vi "Default Instrument Setup.vi"(8 "error in (no error)":errorcluster, 11 "VISA resource name":refnum<visa-resource-name>) -> (0 "error out":errorcluster, 3 "VISA resource name out":refnum<visa-resource-name>)   [LabVIEW 2014, in "GRBLMotionCore.lvlib"]
doc: "This Utility VI sends a default command string to the instrument whenever a new VISA session is opened, or the instrument is reset. Use this VI as a subVI for the Initialize and Reset VIs. Altering this VI could cause these two VIs to operate incorrectly."
uses:
  <instrlib>/GRBL/GRBLMotionCore.lvlib
panel:
  out "Array":string[](array[string])
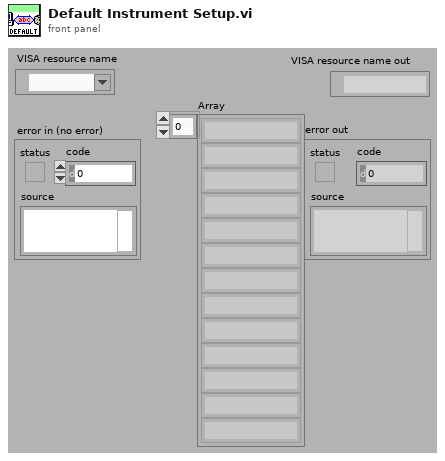
[diagram p1: front panel]
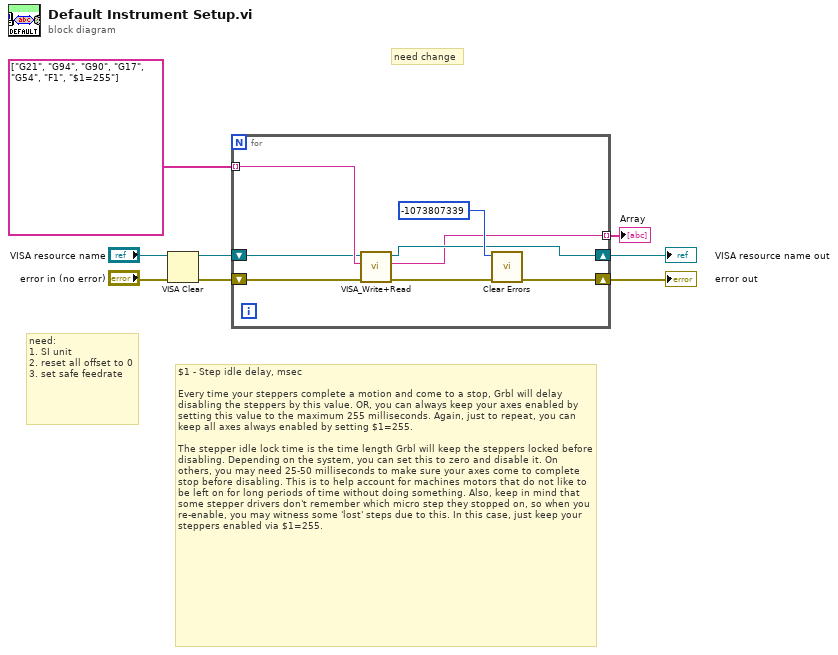
[diagram p0: block diagram]
diagram:
  # "$1 - Step idle delay, msec\n\nEvery time your steppers complete a motion and come to a stop, Grbl will delay disabling the steppers by this value. OR, you can always keep your axes enabled by setting this value to the maximum 255 milliseconds. Again, just to repeat, you can keep all axes always enabled by setting $1=255.\n\nThe stepper idle lock time is the time length Grbl will keep the steppers locked before disabling. Depending on the system, you can set this to zero and disable it. On others, you may need 25-50 milliseconds to make sure your axes come to complete stop before disabling. This is to help account for machines motors that do not like to be left on for long periods of time without doing something. Also, keep in mind that some stepper drivers don't remember which micro step they stopped on, so when you re-enable, you may witness some 'lost' steps due to this. In this case, just keep your steppers enabled via $1=255."
  # "need change"
  # "need:\n1. SI unit\n2. reset all offset to 0\n3. set safe feedrate"
  n1 = VISA Clear(VISA resource name="VISA resource name", error in (no error)="error in (no error)") -> (VISA resource name out=w3:refnum<visa-resource-name>, error out=w2:errorcluster)
  n2 = for {
    tunnel: string[] ["G21", "G94", "G90", "G17", "G54", "F1", "$1=255"] -> [w16] mode=indexing
    shift-right: [w12] -> w7
    shift-left: w3 -> [w13]
    shift-right: [w15] -> w6
    shift-left: w2 -> [w9]
    tunnel: [w10] -> w4 mode=indexing
    n3 = call <instrlib>:"VISA_Write+Read.vi"("error in (no error)"=w9, "Write Buffer"=w16, "VISA resource name"=w13) -> ("error out"=w11:errorcluster, "readout"=w10:string, "VISA resource name out"=w12:refnum<visa-resource-name>)  [unwired: 6 in]
    n4 = call <vilib>:"Clear Errors.vi"("error in (no error)"=w11, "specific error code to clear (0: all)"=-1073807339) -> ("error out"=w15:errorcluster)  [unwired: 4 in, 1 out]
  }
  "error out" <- w6
  "VISA resource name out" <- w7
  "Array" <- w4
